vi "motor_check.vi"() -> ()   [LabVIEW 2013]
uses:
  <vilib>/NXT/Block Support/NXT_InputPort.ctl
  <vilib>/NXT/Block Support/NXT_OutputPort.ctl
  <vilib>/NXT/Dual Mode Library/Sensors/EV3_Gyro_Reset.vi
  <vilib>/NXT/Dual Mode Library/Waits/Wait_Num.vi
  <vilib>/NXT/NXTIO Xnodes/NXTIONodeSubVIs/NXTMoveMotors.vi
  <vilib>/NXT/NXTIO Xnodes/NXTIONodeSubVIs/NXTStopMotors.vi
  <vilib>/NXT/NXTIO Xnodes/NXTIONodeSubVIs/LEGOResetMotors.vi
  <vilib>/NXT/Dual Mode Library/Sensors/Touch_Pressed.vi
  <vilib>/NXT/Dual Mode Library/Sensors/EV3_Gyro_Angle.vi
  <vilib>/NXT/NXTIO Xnodes/NXTIONodeSubVIs/LEGOMotorStatus.vi
  <vilib>/NXT/NXTIO Xnodes/AddressXNode/NXTIOAddress.xnode
  <vilib>/NXT/Subs/LVHSConnector.ctl
  <vilib>/NXT/NXTIO Xnodes/NXTIOXNode/NXTIO.xnode
  <vilib>/NXT/LegoClasses/BrickReference/BrickReference.lvclass
panel:
  in  "File Path":path
  in  "OK Button 4":bool
  in  "OK Button 3":bool
  in  "OK Button 2":bool
  in  "OK Button":bool
  in  "devider":i32=250
  in  "stop":bool
  # "here put the file path"
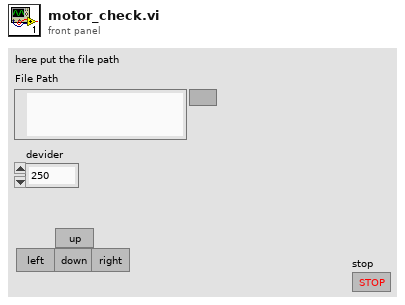
[diagram p1: front panel]
types:
  T1 = typedef "NXT_InputPort.ctl" = u32
  T2 = typedef "NXT_OutputPort.ctl" = u8
  T3 = typedef "LVHSConnector.ctl" = refnum<class "BrickReference.lvclass">
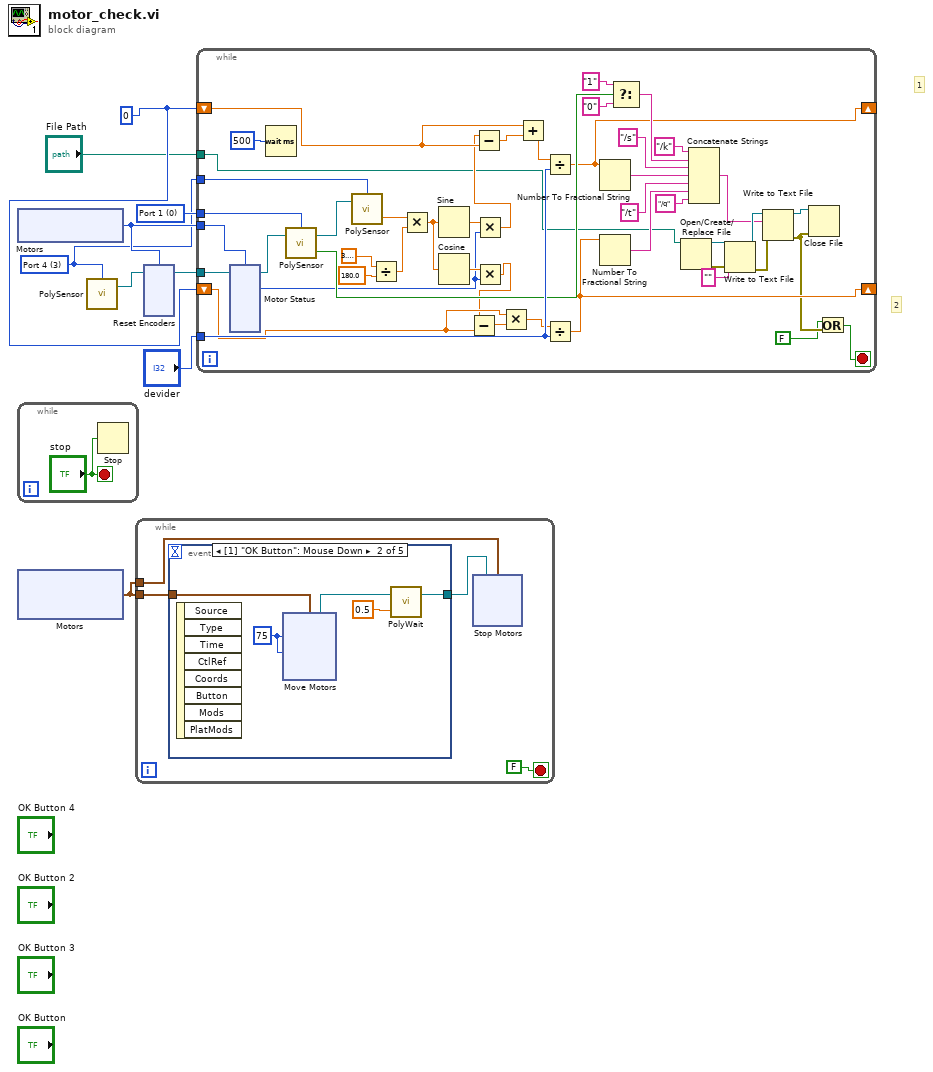
[diagram p0: block diagram]
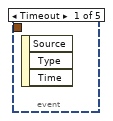
[diagram p2: hidden frame]
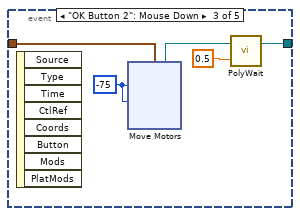
[diagram p3: hidden frame]
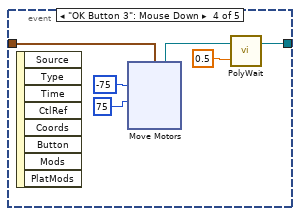
[diagram p4: hidden frame]
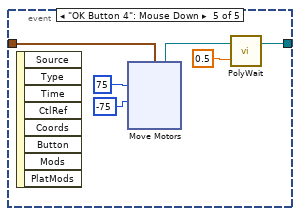
[diagram p5: hidden frame]
diagram:
  w2 = 0
  w5 = T1 3 items=["Port 1", "Port 2", "Port 3", "Port 4"] ("Port (Port 1)")
  w6 = T1 0 items=["Port 1", "Port 2", "Port 3", "Port 4"] ("Port (Port 1)")
  # "2"
  # "1"
  n1 = xnode "Motors"() -> ("Motor"=w9:T2)
  n2 = while {
    stop <- "stop" stop-if-true
    n3 = Stop(stop? (T)="stop") -> ()
  }
  n4 = xnode "Motors"() -> ("Motor"=w3:cluster{"Port":T2, "Port":T2})
  n5 = call-poly <vilib>:"PolySensor.vi"("Port (Port 1)"=w5) -> ("NXT/EV3"=w4:T3)  [unwired: 3 in]
  n6 = while {
    tunnel: w3 -> [w13]
    tunnel: w3 -> [w12]
    stop <- FALSE stop-if-true
    n7 = event shown="[1] \"OK Button\": Mouse Down" {
      selector: _ -> [_ _ _ _ _]
      dyn-events: _ -> [_ _ _ _ _]
      timeout: _ -> [_ _ _ _ _]
      tunnel: [_ w20 w33 w47 w61] -> w14
      tunnel: w13 -> [_ w24 w37 w51 w65]
      event Timeout {
        n8 = event-data() -> ()  [unwired: 1 in, 3 out]
      }
      event "OK Button": Mouse Down {
        w23 = i8 75 ("Power/Speed 1")
        n9 = event-data() -> ()  [unwired: 1 in, 8 out]
        n10 = xnode "Move Motors"("Power/Speed 2"=w23, "Power/Speed 1"=w23, "Motors"=w24) -> ("NXT/EV3"=w21:T3)  [unwired: 1 in]
        n11 = call-poly <vilib>:"PolyWait.vi"("Time (1 sec)"=sgl 0.5, "NXT/EV3"=w21) -> ("NXT/EV3"=w20:T3)  [unwired: 2 in]
      }
      event "OK Button 2": Mouse Down {
        w36 = i8 -75 ("Power/Speed 1")
        n12 = event-data() -> ()  [unwired: 1 in, 8 out]
        n13 = xnode "Move Motors"("Power/Speed 2"=w36, "Power/Speed 1"=w36, "Motors"=w37) -> ("NXT/EV3"=w34:T3)  [unwired: 1 in]
        n14 = call-poly <vilib>:"PolyWait.vi"("Time (1 sec)"=sgl 0.5, "NXT/EV3"=w34) -> ("NXT/EV3"=w33:T3)  [unwired: 2 in]
      }
      event "OK Button 3": Mouse Down {
        n15 = event-data() -> ()  [unwired: 1 in, 8 out]
        n16 = xnode "Move Motors"("Power/Speed 2"=i8 75, "Power/Speed 1"=i8 -75, "Motors"=w51) -> ("NXT/EV3"=w48:T3)  [unwired: 1 in]
        n17 = call-poly <vilib>:"PolyWait.vi"("Time (1 sec)"=sgl 0.5, "NXT/EV3"=w48) -> ("NXT/EV3"=w47:T3)  [unwired: 2 in]
      }
      event "OK Button 4": Mouse Down {
        n18 = event-data() -> ()  [unwired: 1 in, 8 out]
        n19 = xnode "Move Motors"("Power/Speed 2"=i8 -75, "Power/Speed 1"=i8 75, "Motors"=w65) -> ("NXT/EV3"=w60:T3)  [unwired: 1 in]
        n20 = call-poly <vilib>:"PolyWait.vi"("Time (1 sec)"=sgl 0.5, "NXT/EV3"=w60) -> ("NXT/EV3"=w61:T3)  [unwired: 2 in]
      }
    }
    n21 = xnode "Stop Motors"("Motors"=w12, "NXT/EV3"=w14) -> ()  [unwired: 1 out]
  }
  n22 = xnode "Reset Encoders"("Motors"=w9, "NXT/EV3"=w4) -> ("NXT/EV3"=w8:T3)
  n23 = while {
    tunnel: w9 -> [w120]
    tunnel: w8 -> [w115]
    tunnel: "devider" -> [w113]
    tunnel: w6 -> [w112]
    tunnel: w5 -> [w105]
    shift-right: [w94] -> _
    shift-left: w2 -> [w92]
    shift-right: [w85] -> _
    shift-left: w2 -> [w88]
    tunnel: "File Path" -> [w82]
    stop <- w74 stop-if-true
    n24 = xnode "Motor Status"("Motors"=w120, "NXT/EV3"=w115) -> ("Position 1"=w101:i32, "NXT/EV3"=w111:T3)  [unwired: 1 out]
    n25 = Wait (ms)(milliseconds to wait=u32 500) -> ()  [unwired: 1 out]
    n26 = call-poly <vilib>:"PolySensor.vi"("NXT/EV3"=w111, "Port (Port 1)"=w112) -> ("Yes / No"=w110:bool, "NXT/EV3"=w104:T3)  [unwired: 1 in]
    n27 = call-poly <vilib>:"PolySensor.vi"("NXT/EV3"=w104, "Port (Port 1)"=w105) -> ("Degrees"=w99:sgl)  [unwired: 1 in, 1 out]
    n28 = Divide(x=3.141592653589793, y=180.0 ("x")) -> (x/y=w98:dbl)
    n29 = Multiply(x=w99, y=w98) -> (x*y=w97:dbl)
    n30 = Sine(x=w97) -> (sin(x)=w103:dbl)
    n31 = Cosine(x=w97) -> (cos(x)=w102:dbl)
    n32 = Multiply(x=w103, y=w101) -> (x*y=w91:dbl)
    n33 = Subtract(x=w91, y=w92) -> (x-y=w93:dbl)
    n34 = Multiply(x=w102, y=w101) -> (x*y=w87:dbl)
    n35 = Subtract(x=w87, y=w88) -> (x-y=w89:dbl)
    n36 = Multiply(x=w88, y=w89) -> (x*y=w86:dbl)
    n37 = Add(x=w92, y=w93) -> (x+y=w90:dbl)
    n38 = Divide(x=w90, y=w113) -> (x/y=w94:dbl)
    n39 = Divide(x=w86, y=w113) -> (x/y=w85:dbl)
    n40 = Number To Fractional String(number=w94) -> (F-format string=w117:string)  [unwired: 3 in]
    n41 = Number To Fractional String(number=w85) -> (F-format string=w116:string)  [unwired: 3 in]
    n42 = Select(t="1", s=w110, f="0") -> (s? t:f=w107:string)
    n43 = Open/Create/Replace File(file path (use dialog)=w82) -> (refnum out=w81:refnum<file>, error out=w84:errorcluster)  [unwired: 5 in, 1 out]
    n44 = Concatenate Strings("/k" ("string"), w107, "/s" ("string"), w117, "/t" ("string"), w116, "/q" ("string")) -> (w77:string)
    n45 = Write to Text File(file (use dialog)=w81, text="", error in=w84) -> (refnum out=w80:refnum<file>, error out=w79:errorcluster)  [unwired: 1 in, 1 out]
    n46 = Write to Text File(file (use dialog)=w80, text=w77, error in=w79) -> (refnum out=w83:refnum<file>, error out=w76:errorcluster)  [unwired: 1 in, 1 out]
    n47 = Close File(refnum=w83, error in=w76) -> ()  [unwired: 2 out]
    n48 = Or(x=FALSE, y=w76) -> (x .or. y?=w74:bool)
  }
